vi "RequestBigData.vi"(8 "error in (no error)":errorcluster, 10 "Bytes":u32, 11 "module in":refnum<class "TesterModule.lvclass">) -> (0 "error out":errorcluster, 3 "module out":refnum<class "TesterModule.lvclass">)   [LabVIEW 2024, in "TesterModule.lvclass"]
uses:
  TesterModule.lvclass
  C:/Github/JQMH/JQMHCore/Module/JQMHModule.lvclass
  TesterModule.lvclass/TesterModule.ctl
  JQMHCore/Module/JQMHModule.lvclass
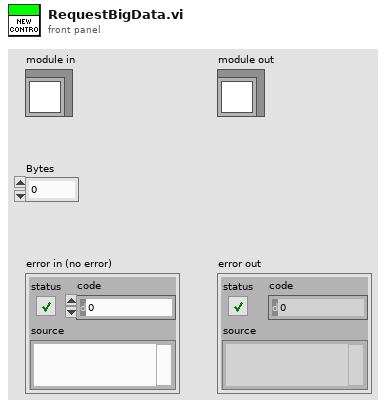
[diagram p1: front panel]
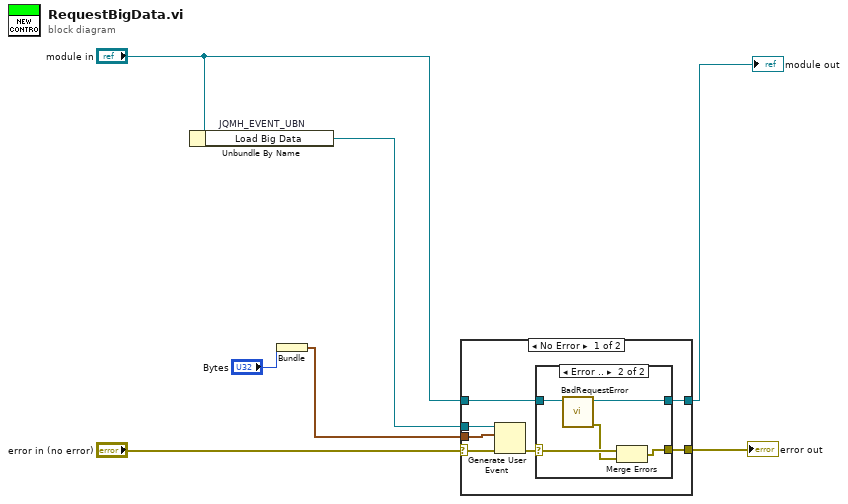
[diagram p0: block diagram]
diagram:
  n1 = Unbundle By Name "JQMH_EVENT_UBN"("module in") -> ("Load Big Data"=w7:refnum<user-event>)
  n2 = Bundle("Bytes"="Bytes") -> (w2:cluster{"Bytes":u32})  [unwired: 1 in]
  n3 = case shown="No Error" "error in (no error)" {
    selector: "error in (no error)" -> [w12 w22]
    tunnel: w7 -> [w14 _]
    tunnel: [w11 w22] -> w5
    tunnel: "module in" -> [w8 w23]
    tunnel: [w10 w23] -> w3
    tunnel: w2 -> [w9 _]
    frame No Error {
      n4 = Generate User Event(user event=w14, event data cluster=w9, error in=w12) -> (error out=w13:errorcluster)  [unwired: 1 in, 1 out]
      n5 = case shown="Error .." w13 {
        selector: w13 -> [w15 w21]
        tunnel: [w15 w20] -> w11
        tunnel: w8 -> [w16 w17]
        tunnel: [w16 w19] -> w10
        frame No Error {
        }
        frame Error {
          n6 = call "BadRequestError.vi"("JQMHModule in"=w17) -> ("error out"=w18:errorcluster, "JQMHModule out"=w19:refnum<class "TesterModule.lvclass">)  [unwired: 9 in]
          n7 = Merge Errors(w21, w18) -> (w20:errorcluster)
        }
      }
    }
    frame Error {
    }
  }
  "error out" <- w5
  "module out" <- w3
